vi "LSCI332VisaRW.vi"(4 "Délais (0 ms)":u32, 5 "Lecture?(T)":bool=TRUE, 6 "error in (no error)":errorcluster, 7 "Nbcaract":u32=100 caption="Nombre de \ncaractères à lire", 8 "EOS (Aucun)":string, 9 "ChaineCom":string caption="Chaîne de commande", 10 "VISA Rsrc":refnum<visa-resource-name>="GPIB0::12::INSTR") -> (0 "error out":errorcluster, 1 "Count out":u32=44 caption="Nombre de caractères lus", 2 "ChaineRep":string caption="Chaîne de réponse", 3 "VISA Rsrc Out":refnum<visa-resource-name>="GPIB0::12::INSTR")   [LabVIEW 2012]
doc: "Ce VI envoie des commande d'écriture et de lecture VISA à l'appareil GPIB. Il permet de ne pas séparer un question de sa réponse. Pour que cela fonctionne toute lecture d'un instrument doit se faire par ce VI."
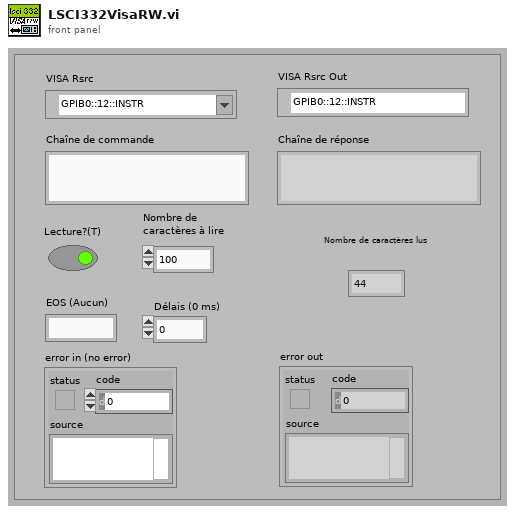
[diagram p1: front panel]
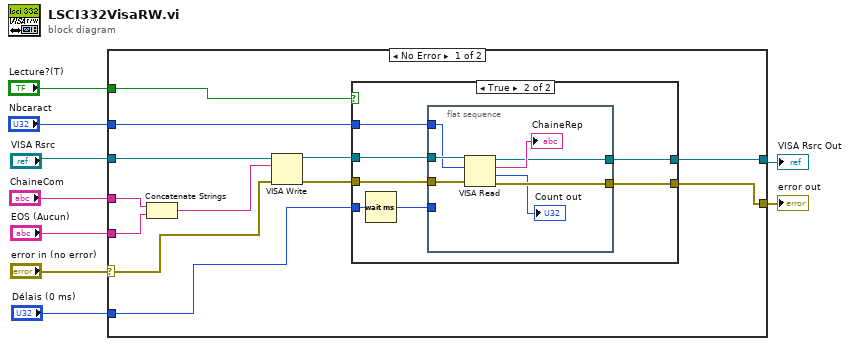
[diagram p0: block diagram]
diagram:
  n1 = case shown="No Error" "error in (no error)" {
    selector: "error in (no error)" -> [w15 w39]
    tunnel: "VISA Rsrc" -> [w16 w38]
    tunnel: [w21 w38] -> w1
    tunnel: "ChaineCom" -> [w20 _]
    tunnel: "EOS (Aucun)" -> [w19 _]
    tunnel: "Délais (0 ms)" -> [w12 _]
    tunnel: "Nbcaract" -> [w11 _]
    tunnel: "Lecture?(T)" -> [w10 _]
    tunnel: [w17 w39] -> w3
    frame No Error {
      n2 = Concatenate Strings(w20, w19) -> (w18:string)
      n3 = VISA Write(VISA resource name=w16, write buffer=w18, error in (no error)=w15) -> (VISA resource name out=w14:refnum<visa-resource-name>, error out=w13:errorcluster)  [unwired: 1 out]
      n4 = case shown="True" w10 {
        tunnel: w14 -> [w23 w30]
        tunnel: [w23 w29] -> w21
        tunnel: w13 -> [w22 w28]
        tunnel: [w22 w27] -> w17
        tunnel: w11 -> [_ w26]
        tunnel: w12 -> [_ w25]
        frame False {
        }
        frame True {
          n5 = Wait (ms)(milliseconds to wait=w25) -> (millisecond timer value=w24:u32)
          n6 = flat-sequence {
            tunnel: [w33] -> w27
            tunnel: [w35] -> w29
            tunnel: w30 -> [w37]
            tunnel: w28 -> [w34]
            tunnel: w26 -> [w31]
            tunnel: w24 -> [_]
            frame #0 {
              n7 = VISA Read(VISA resource name=w37, byte count=w31, error in (no error)=w34) -> (VISA resource name out=w35:refnum<visa-resource-name>, read buffer=→"ChaineRep":string, return count=→"Count out":u32, error out=w33:errorcluster)
            }
          }
        }
      }
    }
    frame Error {
    }
  }
  "error out" <- w3
  "VISA Rsrc Out" <- w1
